vi "Get DAQ Settings.vi"(8 "error in (no error)":errorcluster, 10 "Physical Chan Array":i32[](array[numeric]), 11 "Device Ref in":T1 format="%.0x") -> (0 "error out":errorcluster, 2 "DAQ Config Data":T2, 3 "Device Ref Out":T1 format="%.0x")   [LabVIEW 2020, in "Waveform Analog Output Engine.lvlib"]
doc: "Reads all of the DAQ configuration properties from the custom device"
uses:
  Waveform Analog Output Engine.lvlib
  <vilib>/NI VeriStand/Custom Device API/Custom Device Item Ref.ctl
  DAQ Config Data.ctl
  Shared/Constants.vi
  <vilib>/NI VeriStand/Custom Device API/Get Item Property (String).vi
  <vilib>/NI VeriStand/Custom Device API/Get Item Property (Double).vi
  <vilib>/NI VeriStand/Custom Device API/Get Item Property (U32).vi
  <vilib>/NI VeriStand/Custom Device API/Get Item Property (I32).vi
  <vilib>/NI VeriStand/Custom Device API/Custom Device API.lvlib
  Shared/Waveform Analog Output Shared.lvlib
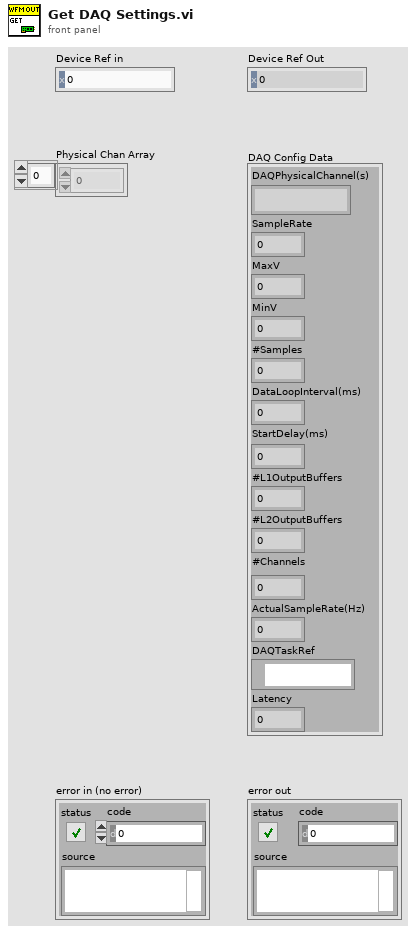
[diagram p1: front panel]
types:
  T1 = typedef "Custom Device API.lvlib/Custom Device Item Ref.ctl" = u64
  T2 = typedef "Waveform Analog Output Engine.lvlib/DAQ Config Data.ctl" = cluster{"DAQPhysicalChannel(s)":string, "SampleRate":dbl, "MaxV":dbl, "MinV":dbl, "#Samples":dbl, "DataLoopInterval(ms)":u32, "StartDelay(ms)":dbl, "#L1OutputBuffers":i32, "#L2OutputBuffers":i32, "#Channels":i32, "ActualSampleRate(Hz)":dbl, "DAQTaskRef":refnum<k21>, "Latency":dbl}
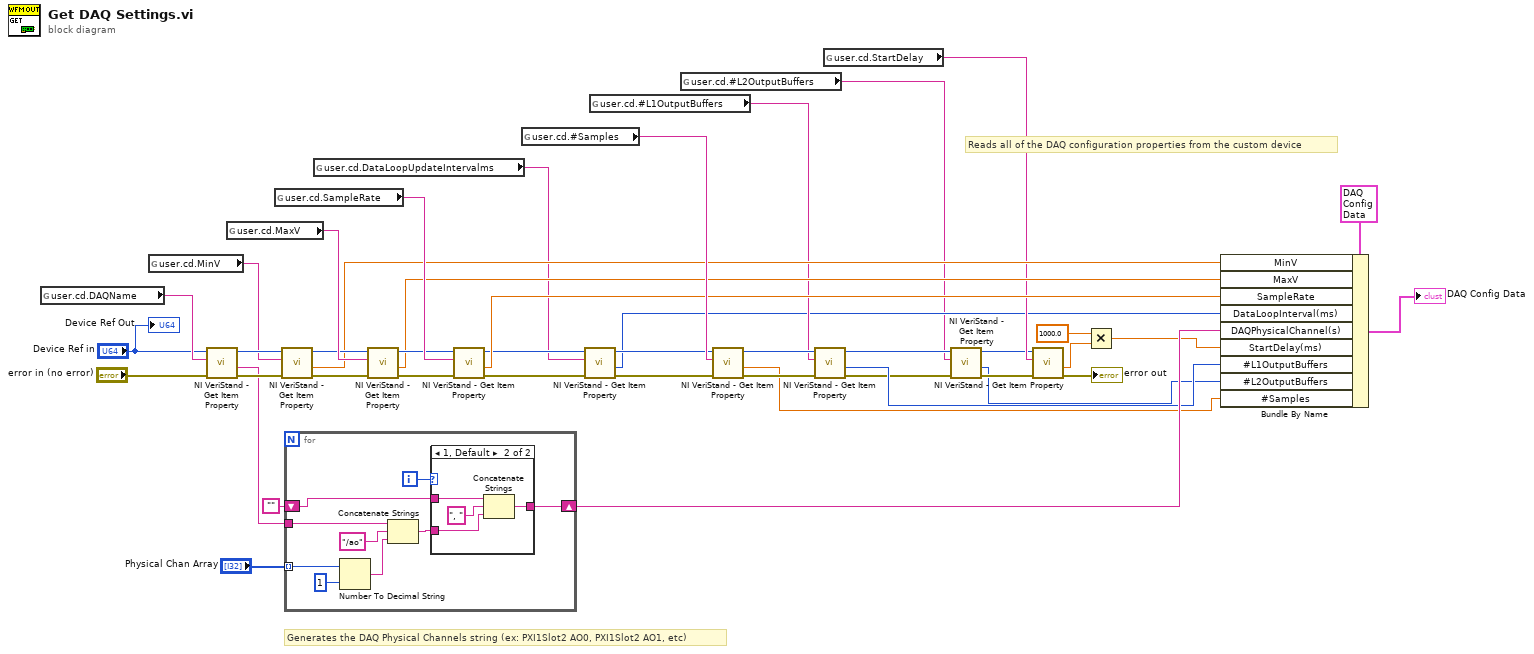
[diagram p0: block diagram]
diagram:
  # "Generates the DAQ Physical Channels string (ex: PXI1Slot2 AO0, PXI1Slot2 AO1, etc)"
  # "Reads all of the DAQ configuration properties from the custom device"
  n1 = global read "Constants.vi" "user.cd.DAQName"() -> (w42:string)
  n2 = global read "Constants.vi" "user.cd.MinV"() -> (w33:string)
  n3 = call-poly <vilib>:"NI VeriStand - Get Item Property.vi"("error in (no error)"="error in (no error)", "Property Name"=w42, "Item Ref in"="Device Ref in") -> ("error out"=w39:errorcluster, "Value"=w30:string, "Item Ref out"=w38:T1)  [unwired: 5 in, 1 out]
  n4 = global read "Constants.vi" "user.cd.MaxV"() -> (w34:string)
  n5 = global read "Constants.vi" "user.cd.SampleRate"() -> (w37:string)
  n6 = call-poly <vilib>:"NI VeriStand - Get Item Property.vi"("error in (no error)"=w39, "Property Name"=w33, "Item Ref in"=w38) -> ("error out"=w32:errorcluster, "Value"=w27:dbl, "Item Ref out"=w31:T1)  [unwired: 5 in, 1 out]
  n7 = for {
    tunnel: w30 -> [w51]
    shift-right: [w46] -> w24
    shift-left: "" -> [w45]
    tunnel: "Physical Chan Array" -> [w50] mode=indexing
    i -> [w53]
    n8 = Number To Decimal String(number=w50, width (-)=i16 1) -> (decimal integer string=w48:string)
    n9 = Concatenate Strings(w51, "/ao" ("string"), w48) -> (w47:string)
    n10 = case shown="1, Default" w53 {
      tunnel: w47 -> [w54 w57]
      tunnel: [w54 w56] -> w46
      tunnel: w45 -> [_ w55]
      frame 0 {
      }
      frame 1, Default {
        n11 = Concatenate Strings(w55, ", " ("string"), w57) -> (w56:string)
      }
    }
  }
  n12 = global read "Constants.vi" "user.cd.DataLoopUpdateIntervalms"() -> (w8:string)
  n13 = call-poly <vilib>:"NI VeriStand - Get Item Property.vi"("error in (no error)"=w32, "Property Name"=w34, "Item Ref in"=w31) -> ("error out"=w36:errorcluster, "Value"=w26:dbl, "Item Ref out"=w35:T1)  [unwired: 5 in, 1 out]
  n14 = call-poly <vilib>:"NI VeriStand - Get Item Property.vi"("error in (no error)"=w36, "Property Name"=w37, "Item Ref in"=w35) -> ("error out"=w11:errorcluster, "Value"=w25:dbl, "Item Ref out"=w12:T1)  [unwired: 5 in, 1 out]
  n15 = global read "Constants.vi" "user.cd.#Samples"() -> (w29:string)
  n16 = call-poly <vilib>:"NI VeriStand - Get Item Property.vi"("error in (no error)"=w11, "Property Name"=w8, "Item Ref in"=w12) -> ("error out"=w10:errorcluster, "Value"=w7:u32, "Item Ref out"=w9:T1)  [unwired: 5 in, 1 out]
  n17 = global read "Constants.vi" "user.cd.#L1OutputBuffers"() -> (w16:string)
  n18 = global read "Constants.vi" "user.cd.#L2OutputBuffers"() -> (w1:string)
  n19 = call-poly <vilib>:"NI VeriStand - Get Item Property.vi"("error in (no error)"=w10, "Property Name"=w29, "Item Ref in"=w9) -> ("error out"=w17:errorcluster, "Value"=w13:dbl, "Item Ref out"=w18:T1)  [unwired: 5 in, 1 out]
  n20 = call-poly <vilib>:"NI VeriStand - Get Item Property.vi"("error in (no error)"=w17, "Property Name"=w16, "Item Ref in"=w18) -> ("error out"=w4:errorcluster, "Value"=w14:i32, "Item Ref out"=w6:T1)  [unwired: 5 in, 1 out]
  n21 = global read "Constants.vi" "user.cd.StartDelay"() -> (w21:string)
  n22 = call-poly <vilib>:"NI VeriStand - Get Item Property.vi"("error in (no error)"=w4, "Property Name"=w1, "Item Ref in"=w6) -> ("error out"=w3:errorcluster, "Value"=w2:i32, "Item Ref out"=w5:T1)  [unwired: 5 in, 1 out]
  n23 = call-poly <vilib>:"NI VeriStand - Get Item Property.vi"("error in (no error)"=w3, "Property Name"=w21, "Item Ref in"=w5) -> ("error out"=→"error out":errorcluster, "Value"=w20:dbl)  [unwired: 5 in, 2 out]
  n24 = Multiply(x=1000.0, y=w20) -> (x*y=w15:dbl)
  n25 = Bundle By Name(cluster=T2 {"DAQPhysicalChannel(s)"="", "SampleRate"=0.0, "MaxV"=0.0, "MinV"=0.0, "#Samples"=0.0, "DataLoopInterval(ms)"=0, "StartDelay(ms)"=0.0, "#L1OutputBuffers"=0, "#L2OutputBuffers"=0, "#Channels"=0, "ActualSampleRate(Hz)"=0.0, "DAQTaskRef"="", "Latency"=0.0} ("DAQ Config Data"), "MinV"=w27, "MaxV"=w26, "SampleRate"=w25, "DataLoopInterval(ms)"=w7, "DAQPhysicalChannel(s)"=w24, "StartDelay(ms)"=w15, "#L1OutputBuffers"=w14, "#L2OutputBuffers"=w2, "#Samples"=w13) -> (→"DAQ Config Data":T2)
  "Device Ref Out" <- "Device Ref in"
